vi "Parse File.vi"(7 "Paths":string[](array[string]), 8 "error in (no error)":errorcluster, 10 "YAML File Path":path, 11 "YAML Parser in":refnum<class "YAML Parser.lvclass">) -> (0 "error out":errorcluster, 3 "YAML Parser out":refnum<class "YAML Parser.lvclass">)   [LabVIEW 2015, in "YAML Parser.lvclass"]
uses:
  YAML Parser.lvclass
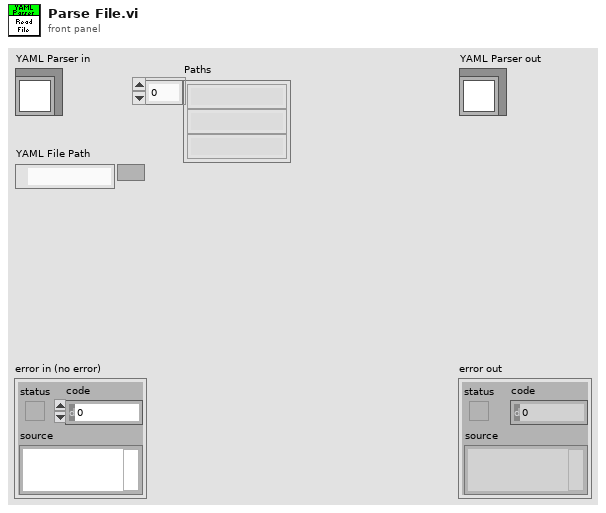
[diagram p1: front panel]
types:
  T1 = enum16{"open", "replace", "create", "open or create", "replace or create", "replace or create with confirmation"}
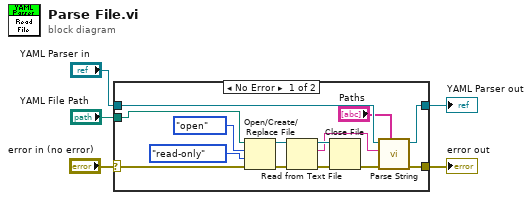
[diagram p0: block diagram]
diagram:
  n1 = case shown="No Error" "error in (no error)" {
    selector: "error in (no error)" -> [w15 w21]
    tunnel: [w10 w21] -> w4
    tunnel: [w8 w20] -> w2
    tunnel: "YAML Parser in" -> [w9 w20]
    tunnel: "YAML File Path" -> [w14 _]
    frame No Error {
      n2 = Open/Create/Replace File(file path (use dialog)=w14, error in=w15, operation (0:open)=T1."open", access (0:read/write)=enum16{"read/write", "read-only", "write-only"}."read-only") -> (refnum out=w19:refnum<file>, error out=w18:errorcluster)  [unwired: 2 in, 1 out]
      n3 = Read from Text File(file (use dialog)=w19, error in=w18) -> (refnum out=w17:refnum<file>, text=w7:string, error out=w16:errorcluster)  [unwired: 2 in, 1 out]
      n4 = Close File(refnum=w17, error in=w16) -> (error out=w11:errorcluster)  [unwired: 1 out]
      n5 = call "Parse String.vi"("Paths"="Paths", "error in (no error)"=w11, "String"=w7, "YAML Parser in"=w9) -> ("error out"=w10:errorcluster, "YAML Parser out"=w8:refnum<class "YAML Parser.lvclass">)  [unwired: 6 in]
    }
    frame Error {
    }
  }
  "error out" <- w4
  "YAML Parser out" <- w2
